vi "2 File IO ex 10 random no Date n Time.vi"() -> ()   [LabVIEW 2016]
panel:
  in  "file path (use dialog)":path=path "C:/Users/Zain/Desktop/test.txt"
  in  "Stop":bool
  # "Temperature"
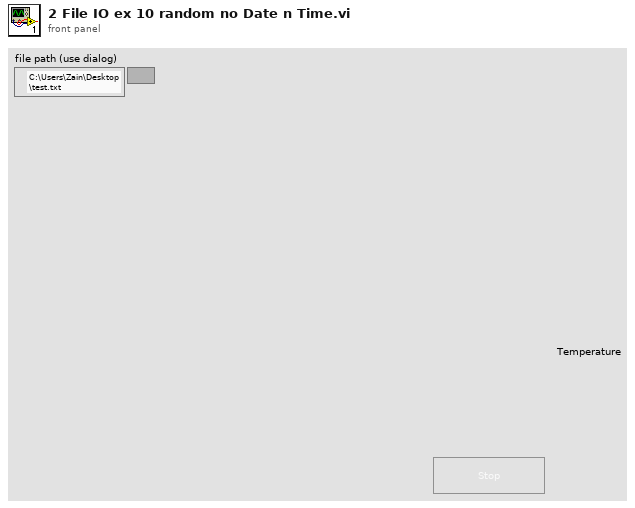
[diagram p1: front panel]
types:
  T1 = enum16{"open", "replace", "create", "open or create", "replace or create", "replace or create with confirmation"}
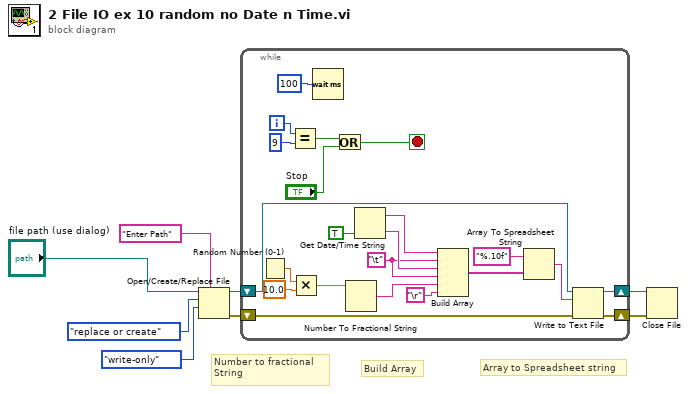
[diagram p0: block diagram]
diagram:
  # "Number to fractional \nString"
  # "Array to Spreadsheet string"
  # "Build Array"
  n1 = Open/Create/Replace File(file path (use dialog)="file path (use dialog)", prompt="Enter Path", operation (0:open)=T1."replace or create", access (0:read/write)=enum16{"read/write", "read-only", "write-only"}."write-only") -> (refnum out=w6:refnum<file>, error out=w5:errorcluster)  [unwired: 1 in, 2 out]
  n2 = while {
    shift-right: [w26] -> w4
    shift-left: w6 -> [w28]
    shift-right: [w25] -> w3
    shift-left: w5 -> [w27]
    i -> [w21]
    stop <- w29 stop-if-true
    w13 = "\t"
    n3 = Random Number (0-1)() -> (number: 0 to 1=w23:dbl)
    n4 = Equal?(x=w21, y=9) -> (x = y?=w19:bool)
    n5 = Multiply(x=w23, y=10.0) -> (x*y=w17:dbl)
    n6 = Wait (ms)(milliseconds to wait=u32 100) -> ()  [unwired: 1 out]
    n7 = Or(x=w19, y="Stop") -> (x .or. y?=w29:bool)
    n8 = Number To Fractional String(number=w17) -> (F-format string=w12:string)  [unwired: 3 in]
    n9 = Get Date/Time String(want seconds? (F)=TRUE) -> (date string=w15:string, time string=w14:string)  [unwired: 2 in]
    n10 = Build Array(w15, w13, w14, w13, w12, "\r") -> (w10:string[])
    n11 = Array To Spreadsheet String(array=w10, 3:"%.10f" ("format string")) -> (spreadsheet string=w9:string)  [unwired: 1 in]
    n12 = Write to Text File(file (use dialog)=w28, text=w9, error in=w27) -> (refnum out=w26:refnum<file>, error out=w25:errorcluster)  [unwired: 1 in, 1 out]
  }
  n13 = Close File(refnum=w4, error in=w3) -> ()  [unwired: 2 out]
